vi "Act1_Histeresis.vi"() -> ()   [LabVIEW 2020]
uses:
  <vilib>/numeric/Random Number (Range) U64.vi
  <vilib>/numeric/sub_Random U32.vi
panel:
  out "Lo que leo":dbl
  out "Histeresis":bool
  out "Rango":bool
  in  "Mínimo":dbl
  in  "Máximo":dbl
  # "Máximo: es el límite máximo"
  # "Mínimo: es el límite mínimo"
  # "Lo que leo: el valor actual arrojado por el número aleatorio."
  # "Indicador \"Rango\": el valor actual se encuentra dentro de los \n                                   límites especificados."
  # "Indicador \"Histéresis\": el indicador es encendido cuando supera \n                                        el rango y se apaga cuando pasa debajo\n                                        del rango."
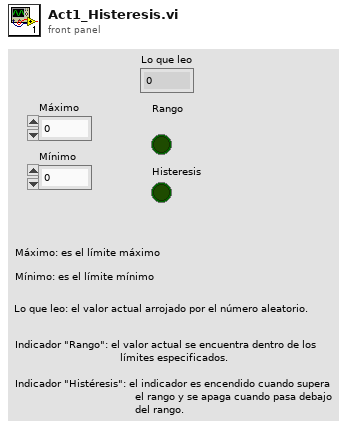
[diagram p1: front panel]
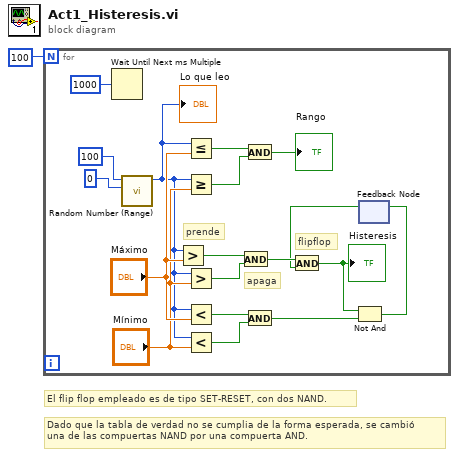
[diagram p0: block diagram]
diagram:
  # "Dado que la tabla de verdad no se cumplia de la forma esperada, se cambió\nuna de las compuertas NAND por una compuerta AND."
  # "El flip flop empleado es de tipo SET-RESET, con dos NAND."
  n1 = for {
    N: 100 -> [_]
    # "flipflop"
    # "apaga"
    # "prende"
    n2 = Wait Until Next ms Multiple(millisecond multiple=u32 1000) -> ()  [unwired: 1 out]
    n3 = call-poly <vilib>:"Random Number (Range).vi"("lower bound (0)"=u64 0, "upper bound (100)"=u64 100) -> ("number"=w2:u64)  [unwired: 9 in]
    "Lo que leo" <- w2
    n4 = Greater?(x=w2, y="Máximo") -> (0:w13:bool)
    n5 = Less Or Equal?(x=w2, y="Máximo") -> (x <= y?=w16:bool)
    n6 = Greater Or Equal?(x=w2, y="Mínimo") -> (x >= y?=w15:bool)
    n7 = Greater?(x=w2, y="Mínimo") -> (0:w5:bool)
    n8 = Less?(x=w2, y="Máximo") -> (x < y?=w11:bool)
    n9 = Less?(x=w2, y="Mínimo") -> (x < y?=w10:bool)
    n10 = And(x=w13, y=w5) -> (x .and. y?=w9:bool)
    n11 = And(x=w16, y=w15) -> (x .and. y?=→"Rango":bool)
    n12 = And(x=w11, y=w10) -> (x .and. y?=w8:bool)
    n13 = feedback #1() -> (w3:bool)  [unwired: 1 in]
    n14 = And(x=w9, y=w3) -> (x .and. y?=w7:bool)
    "Histeresis" <- w7
    n15 = Not And(1:w8, 2:w7) -> (0:w4:bool)
    n16 = feedback-in #1(w4) -> ()
  }
